vi "Abort Logger.vi"(8 "Error In":errorcluster, 11 "TDMS Log In":refnum<class "TDMS Logger.lvclass">) -> (0 "Error Out":errorcluster)   [LabVIEW 2019, in "TDMS Logger.lvlib" / "TDMS Logger.lvclass"]
doc: "This VI will abort the data logger. All data that was not saved and is still in the data logger queue will be discarded.\n\nMaximum time spent in this VI waiting for the asynchronous logging loop to abort is 50ms.\n<b>If that time is not enough then the TDMS file reference might remain open.</b>\n\nTo be sure and safe while stopping the logging please use the <b>Log Rest and Release</b> method."
uses:
  TDMS Logger.lvclass
  _Typedefs/Log Action.ctl
  _Typedefs/Log Message.ctl
  _Typedefs/Data Type.ctl
  TDMS Logger.lvclass/TDMS Logger.ctl
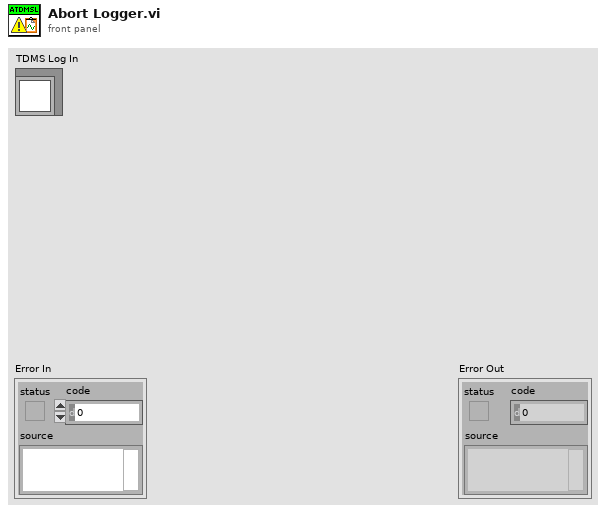
[diagram p1: front panel]
types:
  T1 = typedef "TDMS Logger.lvlib/TDMS Logger.lvclass/Log Action.ctl" = enum16{"Handle Old Files", "Status Update", "Stop", "Log Data", "Initialize"}
  T2 = typedef "TDMS Logger.lvlib/TDMS Logger.lvclass/Log Message.ctl" = cluster{"Log Action":T1, "Variant":variant, "Data Type":T3, "Group Name":string, "Channels Names":string[]}
  T3 = typedef "TDMS Logger.lvlib/TDMS Logger.lvclass/Data Type.ctl" = enum16{"I16", "I8", "String", "U16", "U8", "Waveform", "Double", "Single"}
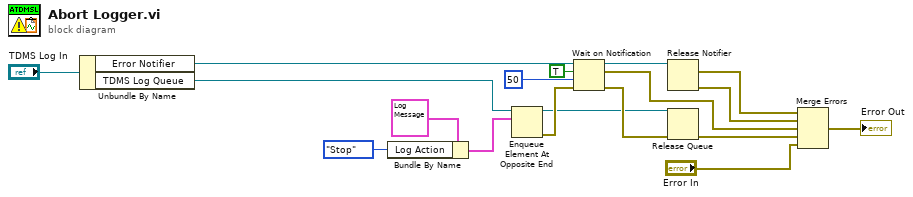
[diagram p0: block diagram]
diagram:
  n1 = Unbundle By Name("TDMS Log In") -> ("Error Notifier"=w17:refnum<notifier>, "TDMS Log Queue"=w2:refnum<queue>)
  n2 = Bundle By Name(cluster=T2 {"Log Action"=enum."Stop", "Variant"=variant, "Data Type"=enum."String", "Group Name"="", "Channels Names"=[]} ("element"), "Log Action"=Log_Action."Stop") -> (w11:T2)
  n3 = Enqueue Element At Opposite End(queue=w2, element=w11) -> (queue out=w4:refnum<queue>, error out=w6:errorcluster)  [unwired: 2 in, 1 out]
  n4 = Wait on Notification(notifier=w17, ignore previous (F)=TRUE, timeout in ms (-1)=50, error in (no error)=w6) -> (notifier out=w9:refnum<notifier>, notification=w3:errorcluster, error out=w5:errorcluster)  [unwired: 1 out]
  n5 = Release Notifier(notifier=w9) -> (last notification=w14:errorcluster, error out=w15:errorcluster)  [unwired: 2 in, 1 out]
  n6 = Release Queue(queue=w4, error in (no error)=w5) -> (error out=w16:errorcluster)  [unwired: 1 in, 2 out]
  n7 = Merge Errors(w14, w15, w3, w16, "Error In") -> (→"Error Out":errorcluster)
